vi "Vendor_Management.vi"() -> ()   [LabVIEW 2023]
panel:
  in  "stop":bool
  in  "Numeric":dbl
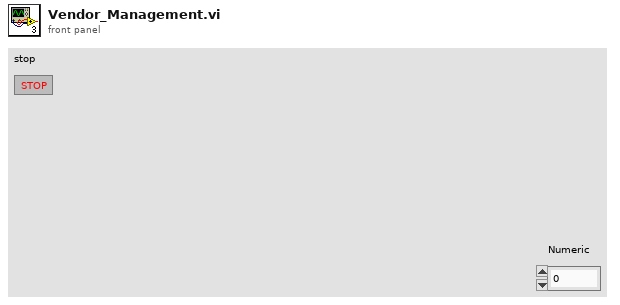
[diagram p1: front panel]
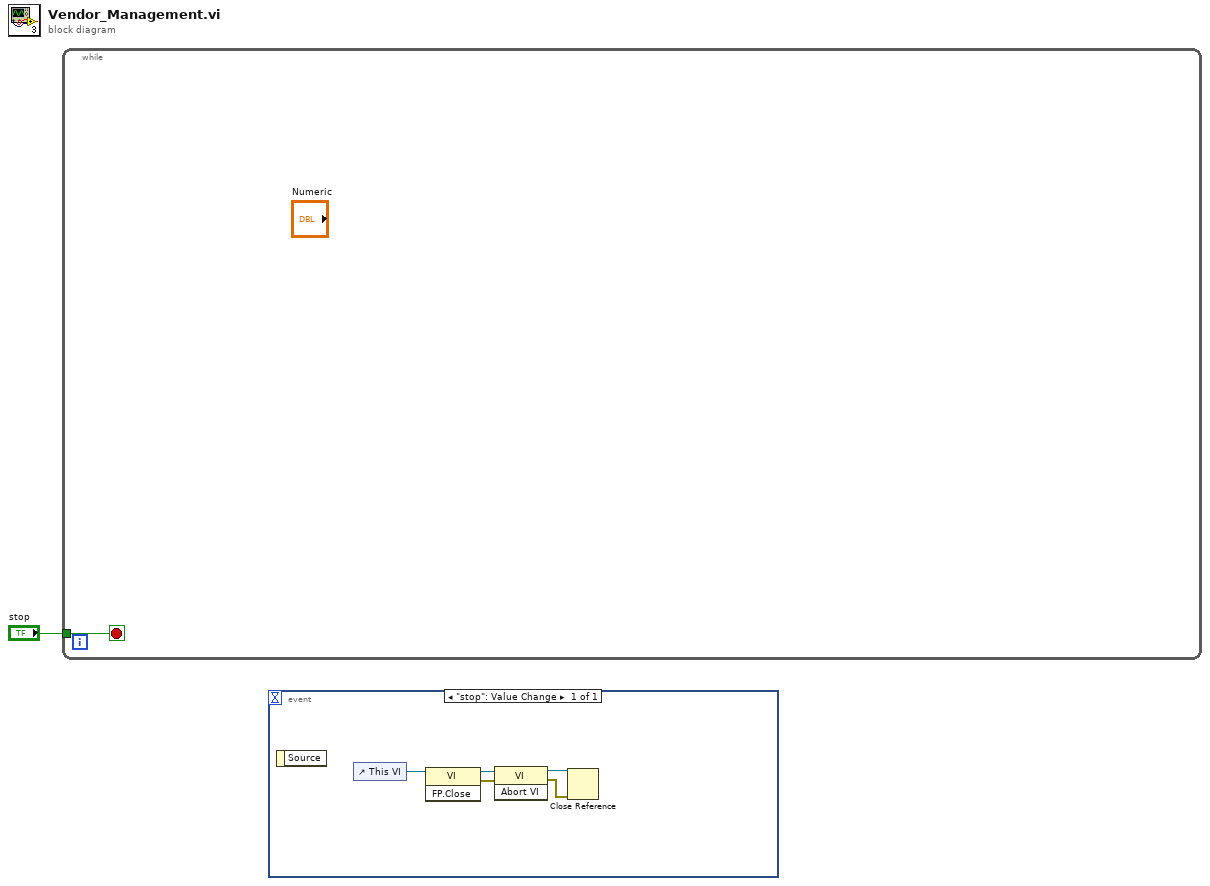
[diagram p0: block diagram]
diagram:
  n1 = while {
    tunnel: "stop" -> [w2]
    stop <- w2 stop-if-true
  }
  n2 = event shown="[0] \"stop\": Value Change" {
    selector: _ -> [_]
    dyn-events: _ -> [_]
    timeout: _ -> [_]
    event "stop": Value Change {
      n3 = event-data() -> ()  [unwired: 1 in, 1 out]
      n4 = control-ref of="This VI"() -> (w7:refnum<vi>)
      n5 = invoke class="VI" method="FP.Close"(reference=w7) -> (reference out=w6:refnum<vi>, error out=w5:errorcluster)  [unwired: 2 in, 1 out]
      n6 = invoke class="VI" method="Abort VI"(reference=w6, error in=w5) -> (reference out=w4:refnum<vi>, error out=w3:errorcluster)  [unwired: 1 in, 1 out]
      n7 = Close Reference(reference=w4, error in (no error)=w3) -> ()  [unwired: 1 out]
    }
  }
